vi "Measure Targets.vi"(5 "Image":T1, 7 "FOV width":dbl, 11 "Unmeasured Targets in":T2[](array[typedef])) -> (3 "Measured Targets out":T2[](array[typedef]))   [LabVIEW 2015]
uses:
  Vision Tote Data.ctl
  <vilib>/vision/Image Controls.llb/IMAQ Image.ctl
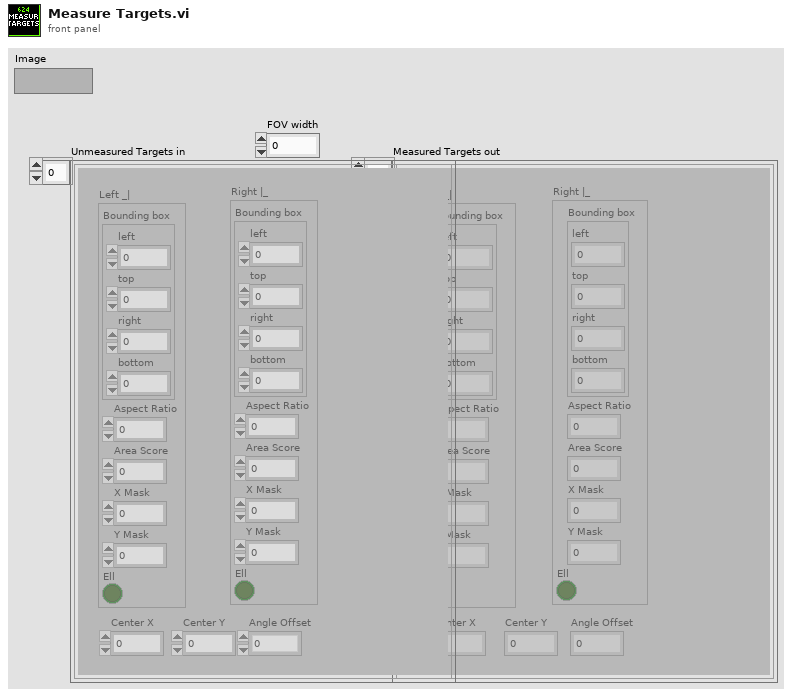
[diagram p1: front panel]
types:
  T1 = typedef "IMAQ Image.ctl" = refnum<image>
  T2 = typedef "Vision Tote Data.ctl" = cluster{"Left _|":cluster{"Bounding box":cluster{"left":dbl, "top":dbl, "right":dbl, "bottom":dbl}, "Aspect Ratio":dbl, "Area Score":dbl, "X Mask":dbl, "Y Mask":dbl, "Ell":bool}, "Right |_":cluster{"Bounding box":cluster{"left":dbl, "top":dbl, "right":dbl, "bottom":dbl}, "Aspect Ratio":dbl, "Area Score":dbl, "X Mask":dbl, "Y Mask":dbl, "Ell":bool}, "Center X":dbl, "Center Y":dbl, "Angle Offset":dbl}
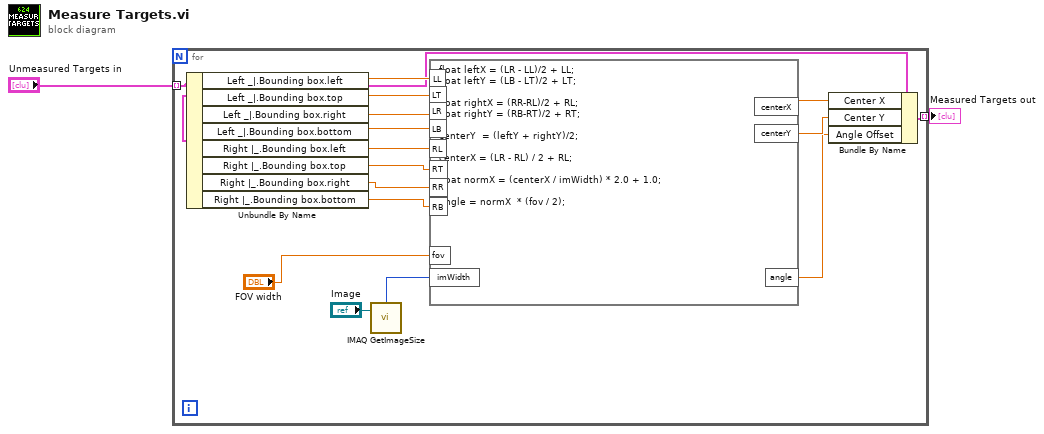
[diagram p0: block diagram]
diagram:
  n1 = for {
    tunnel: "Unmeasured Targets in" -> [w10] mode=indexing
    tunnel: [w8] -> w1 mode=indexing
    n2 = Unbundle By Name(w10) -> ("Left _|.Bounding box.left"=w18:dbl, "Left _|.Bounding box.top"=w17:dbl, "Left _|.Bounding box.right"=w16:dbl, "Left _|.Bounding box.bottom"=w15:dbl, "Right |_.Bounding box.left"=w14:dbl, "Right |_.Bounding box.top"=w13:dbl, "Right |_.Bounding box.right"=w12:dbl, "Right |_.Bounding box.bottom"=w11:dbl)
    n3 = call "IMAQ GetImageSize"("Image"="Image") -> ("X Resolution"=w4:i32)  [unwired: 3 in, 2 out]
    n4 = formula code="float leftX = (LR - LL)/2 + LL;\nfloat leftY = (LB - LT)/2 + LT;\n\nfloat rightX = (RR-RL)/2 + RL;\nfloat rightY = (RB-RT)/2 + RT;\n\ncenterY  = (leftY + rightY)/2; \n\ncenterX = (LR - RL) / 2 + RL;\n\nfloat normX = (centerX / imWidth) * 2.0 + 1.0;\n\nangle = normX  * (fov / 2);"("LL"=w18, "LT"=w17, "LR"=w16, "LB"=w15, "RL"=w14, "RT"=w13, "RR"=w12, "RB"=w11, "fov"="FOV width", "imWidth"=w4) -> ("centerX"=w9:dbl, "centerY"=w6:dbl, "angle"=w5:dbl)
    n5 = Bundle By Name(cluster=w10, "Center X"=w9, "Center Y"=w6, "Angle Offset"=w5) -> (w8:T2)
  }
  "Measured Targets out" <- w1
